vi "LV Image to Jpeg string (Quality) v2.vi"() -> ()   [LabVIEW 2011]
uses:
  System.Drawing
panel:
  out "size":i32
  in  "Quality":u8=100
  in  "JPEG File":path
  out "Jpeg String":string
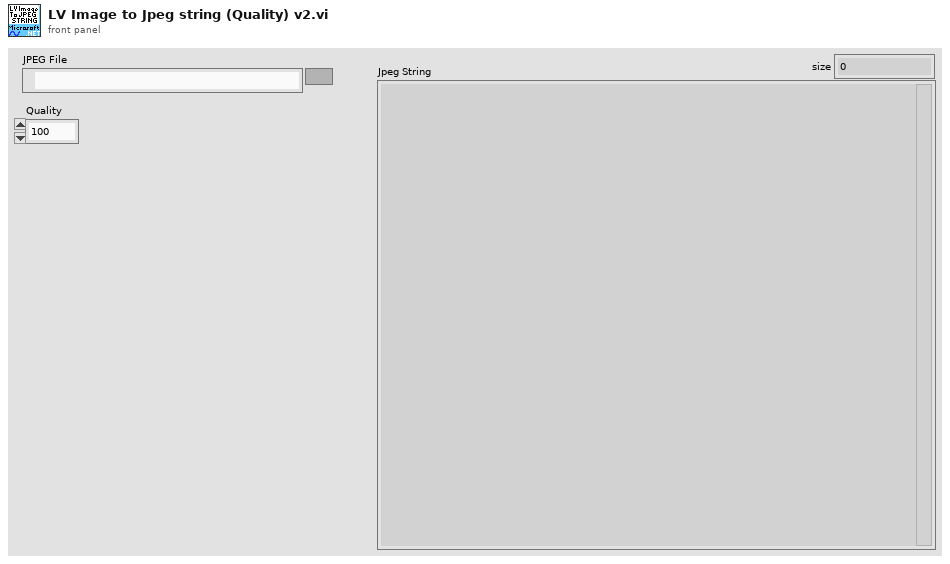
[diagram p1: front panel]
types:
  T1 = typedef "imagedata.ctl" = cluster{"image type":i32, "image depth":i32, "image":u8[], "mask":u8[], "colors":u32[], "Rectangle":cluster{"left":i16, "top":i16, "right":i16, "bottom":i16}}
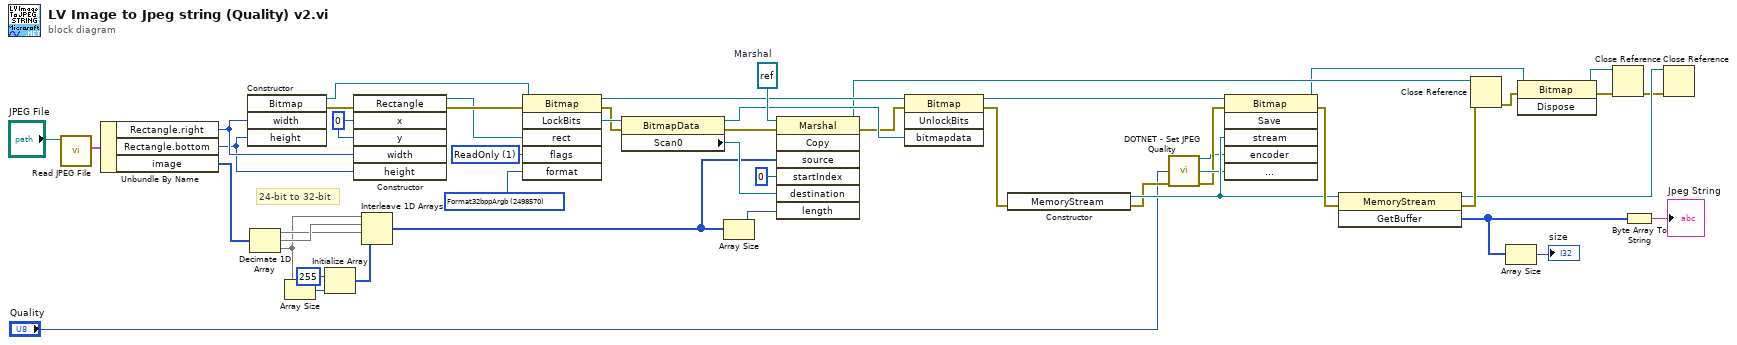
[diagram p0: block diagram]
diagram:
  w34 = refnum<k24> refnum  # Marshal
  w37 = 2498570 items=["DontCare, Undefined"=0, "Max"=15, "Indexed"=65536, "Gdi"=131072, "Format16bppRgb555"=135173, "Format16bppRgb565"=135174, "Format24bppRgb"=137224, "Format32bppRgb"=139273, "Format1bppIndexed"=196865, "Format4bppIndexed"=197634, "Format8bppIndexed"=198659, "Alpha"=262144, "Format16bppArgb1555"=397319, "PAlpha"=524288, "Format32bppPArgb"=925707, "Extended"=1048576, "Format16bppGrayScale"=1052676, "Format48bppRgb"=1060876, "Format64bppPArgb"=1851406, "Canonical"=2097152, "Format32bppArgb"=2498570, "Format64bppArgb"=3424269] ("format")
  w38 = 1 items=["ReadOnly"=1, "WriteOnly"=2, "ReadWrite"=3, "UserInputBuffer"=4] ("flags")
  w45 = 0 ("x")
  # "24-bit to 32-bit"
  n1 = call <vilib>:"Read JPEG File.vi"("path to JPEG file"="JPEG File") -> ("image data"=w47:T1)  [unwired: 8 in, 2 out]
  n2 = Unbundle By Name(w47) -> ("Rectangle.right"=w44:i16, "Rectangle.bottom"=w43:i16, "image"=w8:u8[])
  n3 = constructor class="Bitmap"("width"=w44, "height"=w43) -> (reference out=w41:refnum<k24>, error out=w42:errorcluster)  [unwired: 3 in, 3 out]
  n4 = Decimate 1D Array(w8) -> (w6:u8[], w7:u8[], w4:u8[])
  n5 = Array Size(array=w4) -> (size(s)=w3:i32)
  n6 = Initialize Array(u8 255 ("Quality"), w3) -> (w1:u8[])
  n7 = constructor class="Rectangle"(error in=w42, "x"=w45, "y"=w45, "width"=w44, "height"=w43) -> (reference out=w39:refnum<k24>, error out=w40:errorcluster)  [unwired: 2 in, 5 out]
  n8 = Interleave 1D Arrays(w4, w7, w6, w1) -> (w5:u8[])
  n9 = invoke class="Bitmap" method="LockBits"(reference=w41, error in=w40, "rect"=w39, "flags"=w38, "format"=w37) -> (reference out=w29:refnum<k24>, error out=w35:errorcluster, "LockBits"=w36:refnum<k24>)  [unwired: 1 in, 3 out]
  n10 = property class="BitmapData"(reference=w36, error in=w35) -> (reference out=w28:refnum<k24>, error out=w33:errorcluster, "Scan0"=w31:refnum<k24>)
  n11 = Array Size(array=w5) -> (size(s)=w30:i32)
  n12 = invoke class="Marshal" method="Copy"(reference=w34, error in=w33, "source"=w5, "startIndex"=0, "destination"=w31, "length"=w30) -> (reference out=w23:refnum<k24>, error out=w27:errorcluster)  [unwired: 1 in, 5 out]
  n13 = invoke class="Bitmap" method="UnlockBits"(reference=w29, error in=w27, "bitmapdata"=w28) -> (reference out=w26:refnum<k24>, error out=w25:errorcluster)  [unwired: 1 in, 2 out]
  n14 = constructor class="MemoryStream"(error in=w25) -> (reference out=w16:refnum<k24>, error out=w14:errorcluster)  [unwired: 2 in, 1 out]
  n15 = call "DOTNET - Set JPEG Quality.vi"("Quality"="Quality", "error in (no error)"=w14) -> ("ImageCodecInfo"=w11:refnum<k24>, "EncoderParameters"=w15:refnum<k24>, "error out"=w12:errorcluster)  [unwired: 11 in]
  n16 = invoke class="Bitmap" method="Save"(reference=w26, error in=w12, "stream"=w16, "encoder"=w11, "encoderParams"=w15) -> (reference out=w22:refnum<k24>, error out=w46:errorcluster)  [unwired: 1 in, 4 out]
  n17 = invoke class="MemoryStream" method="GetBuffer"(reference=w16, error in=w46) -> (reference out=w18:refnum<k24>, error out=w24:errorcluster, "GetBuffer"=w10:u8[])  [unwired: 1 in]
  n18 = Close Reference(reference=w23, error in (no error)=w24) -> (error out=w21:errorcluster)
  n19 = Array Size(array=w10) -> (size(s)=→"size":i32)
  n20 = invoke class="Bitmap" method="Dispose"(reference=w22, error in=w21) -> (reference out=w19:refnum<k24>, error out=w20:errorcluster)  [unwired: 1 in, 1 out]
  n21 = Close Reference(reference=w19, error in (no error)=w20) -> (error out=w17:errorcluster)
  n22 = Byte Array To String(unsigned byte array=w10) -> (string=→"Jpeg String":string)
  n23 = Close Reference(reference=w18, error in (no error)=w17) -> ()  [unwired: 1 out]
